vi "drive straight auto.vi"(7 "PID stuff":T1={"K Derivative"=0.000578344411839991, "K Proportional"=0.06728988505411036, "K Integral"=0.0} {"K Integral" scale=0.0..0.1; "K Proportional" scale=0.0..0.1; "K Derivative" scale=0.0..0.1}, 10 "Foward Power":dbl(knob) scale=0.0..1.0, 11 "Foward Distance":dbl) -> ()   [LabVIEW 2011]
uses:
  <vilib>/addons/control/pid/pid.llb/PID (DBL).vi
  <vilib>/addons/control/pid/NI_PID_pid.lvlib
panel:
  out "Waveform Chart":dbl(graph)
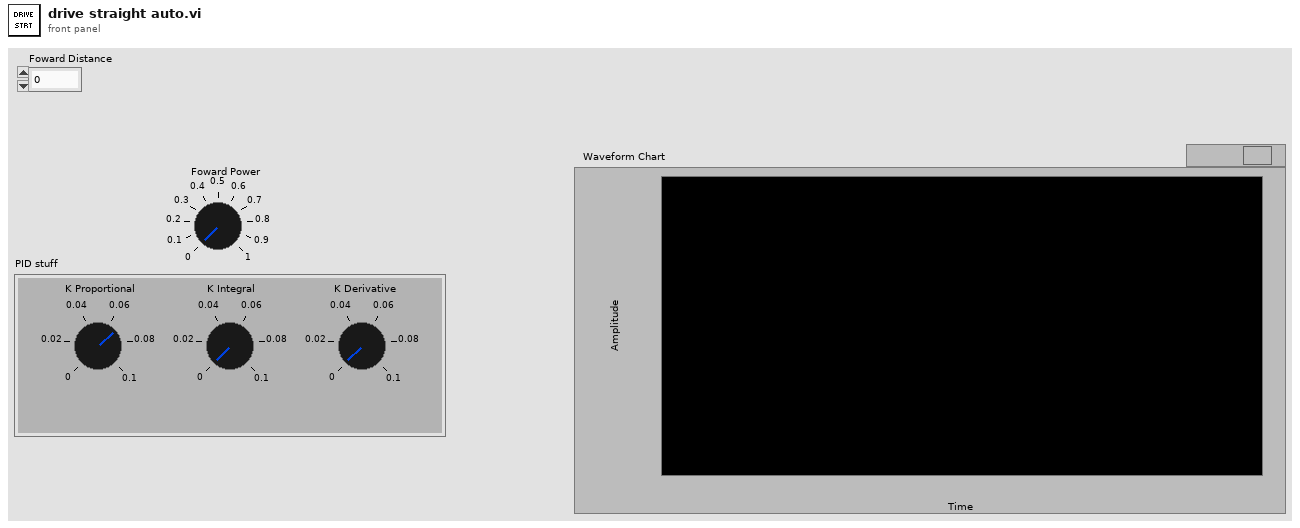
[diagram p1: front panel]
types:
  T1 = cluster{"K Derivative":dbl, "K Proportional":dbl, "K Integral":dbl}
  T2 = typedef "WPI_EncoderDevRef.ctl" = cluster{"DevStatus":errorcluster, "EncoderIndex":T3, "CounterIndex":T4, "DistancePerCount":dbl, "Decoding Type":T5}
  T3 = typedef "FPGA_EncoderIdx.ctl" = enum8{"Enc 0", "Enc 1", "Enc 2", "Enc 3", "Invalid"}
  T4 = typedef "FPGA_CounterCtrSystemIndex.ctl" = enum8{"Ctr 0", "Ctr 1", "Ctr 2", "Ctr 3", "Ctr 4", "Ctr 5", "Ctr 6", "Ctr 7", "Invalid"}
  T5 = typedef "WPI_EncoderType.ctl" = enum16{"1x", "2x", "4x"}
  T6 = typedef "WPI_GyroDevRef.ctl" = cluster{"DevStatus":errorcluster, "Analog Module":T7, "Analog Channel":T8, "Offset":dbl, "Gain (VoltsPerDegree/Second)":dbl}
  T7 = typedef "FPGA_TypedefAnalogModule.ctl" = enum16{"Analog Module 1", "Analog Module 2"}
  T8 = typedef "FPGA_AIChannel.ctl" = enum8{"AI 1", "AI 2", "AI 3", "AI 4", "AI 5", "AI 6", "AI 7", "AI 8", "Invalid"}
  T9 = typedef "WPI_RobotDriveDevRef.ctl" = cluster{"DevStatus":errorcluster, "Motors[]":T10[], "Square Inputs":bool, "Max Output":dbl, "Isochronous":bool}
  T10 = typedef "WPI_MotorControlDeviceRef.ctl" = cluster{"DeviceStatus":errorcluster, "Type":enum16{"PWM", "CAN"}, "PWM":cluster{"Digital Module":T11, "PWM Channel":T12, "DeadBand":T13}, "CAN":cluster{"Device Number":u8, "Control Mode":T14, "Semaphore":T15, "Max Vout":dbl}, "Invert":bool, "TransformRef":T16, "InvTransformRef":T16}
  T11 = typedef "FPGA_TypedefDigitalModule.ctl" = enum16{"Digital Module 1", "Digital Module 2"}
  T12 = typedef "FPGA_DIOPWMChannel.ctl" = enum8{"PWM 1", "PWM 2", "PWM 3", "PWM 4", "PWM 5", "PWM 6", "PWM 7", "PWM 8", "PWM 9", "PWM 10", "Invalid"}
  T13 = typedef "WPI_PWMDeadband.ctl" = cluster{"Name":string, "maxPositivePwm":i32, "minPositivePwm":i32, "centerPwm":i32, "maxNegativePwm":i32, "minNegativePwm":i32, "angularRange":u16}
  T14 = typedef "WPI_CANJaguar_ControlMode.ctl" = enum8{"Percent VBus", "Current", "Speed", "Position", "Voltage"}
  T15 = typedef "Semaphore RefNum" = refnum<k1>
  T16 = typedef "WPI_PWMTransform_ConPane.ctl" = refnum<vi>
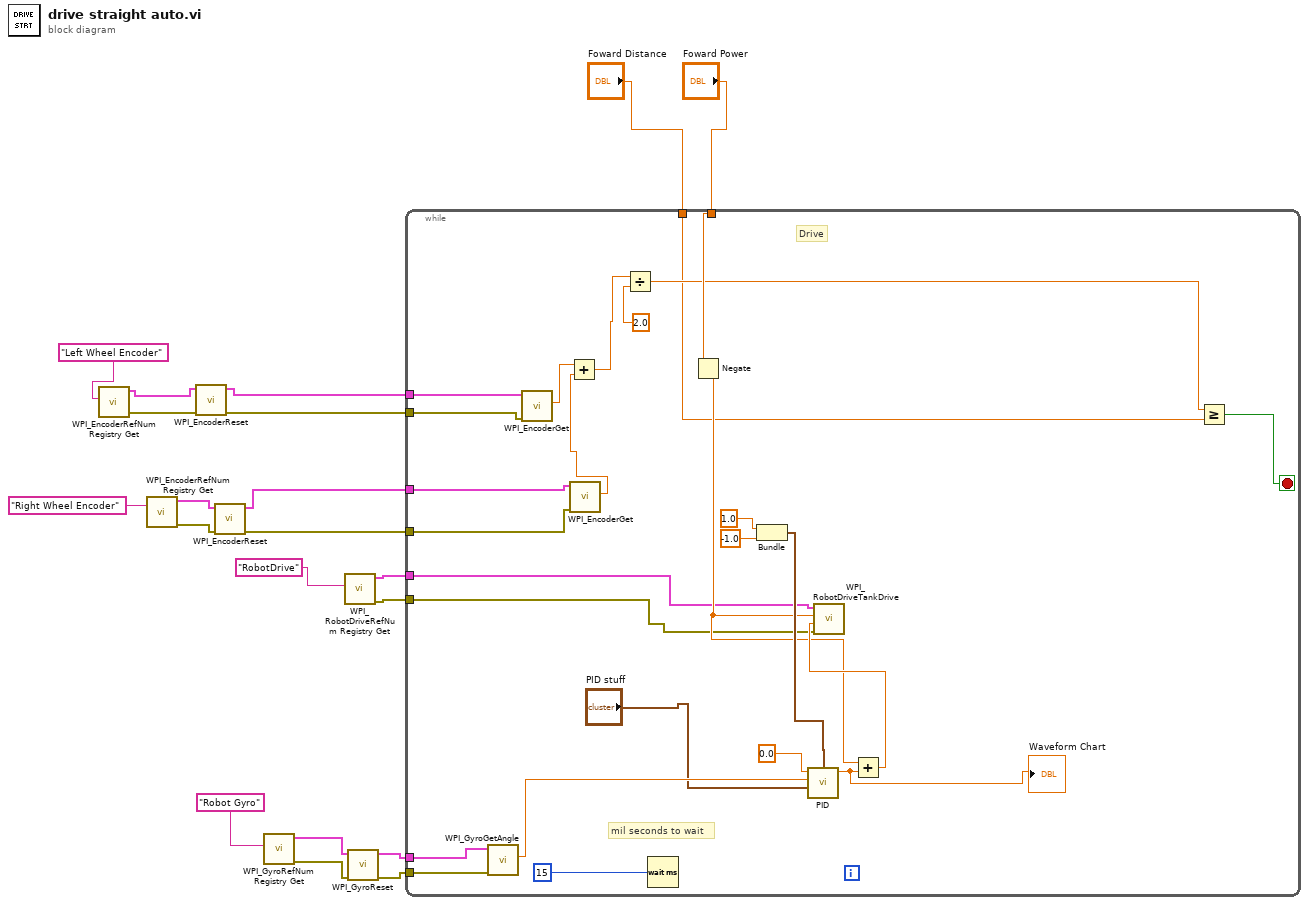
[diagram p0: block diagram]
diagram:
  n1 = call <vilib>:"WPI_EncoderRefNum Registry Get.vi"("refnum name"="Left Wheel Encoder") -> ("error out"=w16:errorcluster, "EncoderDevRef"=w17:T2)  [unwired: 9 in]
  n2 = call <vilib>:"WPI_EncoderRefNum Registry Get.vi"("refnum name"="Right Wheel Encoder") -> ("error out"=w14:errorcluster, "EncoderDevRef"=w15:T2)  [unwired: 9 in]
  n3 = call <vilib>:"WPI_EncoderReset.vi"("error in (no error)"=w16, "EncoderDevRef"=w17) -> ("error out"=w10:errorcluster, "EncoderDevRef"=w11:T2)  [unwired: 8 in]
  n4 = call <vilib>:"WPI_EncoderReset.vi"("error in (no error)"=w14, "EncoderDevRef"=w15) -> ("error out"=w12:errorcluster, "EncoderDevRef"=w13:T2)  [unwired: 8 in]
  n5 = call <vilib>:"WPI_GyroRefNum Registry Get.vi"("refnum name"="Robot Gyro") -> ("error out"=w2:errorcluster, "GyroDevRef"=w3:T6)  [unwired: 9 in]
  n6 = call <vilib>:"WPI_RobotDriveRefNum Registry Get.vi"("refnum name"="RobotDrive") -> ("error out"=w6:errorcluster, "RobotDriveDevRef"=w7:T9)  [unwired: 9 in]
  n7 = call <vilib>:"WPI_GyroReset.vi"("error in (no error)"=w2, "GyroDevRef"=w3) -> ("error out"=w5:errorcluster, "GyroDevRef"=w4:T6)  [unwired: 8 in]
  n8 = while {
    tunnel: "Foward Distance" -> [w21]
    tunnel: "Foward Power" -> [w43]
    tunnel: w13 -> [w30]
    tunnel: w12 -> [w29]
    tunnel: w11 -> [w28]
    tunnel: w10 -> [w27]
    tunnel: w4 -> [w26]
    tunnel: w5 -> [w25]
    tunnel: w7 -> [w24]
    tunnel: w6 -> [w23]
    stop <- w39 stop-if-true
    # "mil seconds to wait"
    # "Drive"
    n9 = call <vilib>:"WPI_GyroGetAngle.vi"("error in (no error)"=w25, "GyroDevRef"=w26) -> ("Angle"=w34:dbl)  [unwired: 6 in, 3 out]
    n10 = call <vilib>:"WPI_EncoderGet.vi"("error in (no error)"=w27, "EncoderDevRef"=w28) -> ("Distance"=w33:dbl)  [unwired: 4 in, 5 out]
    n11 = call <vilib>:"WPI_EncoderGet.vi"("error in (no error)"=w29, "EncoderDevRef"=w30) -> ("Distance"=w35:dbl)  [unwired: 4 in, 5 out]
    n12 = Add(x=w33, y=w35) -> (x+y=w32:dbl)
    n13 = Divide(x=w32, y=2.0) -> (x/y=w37:dbl)
    n14 = Wait (ms)(milliseconds to wait=u32 15) -> ()  [unwired: 1 out]
    n15 = Negate(x=w43) -> (-x=w36:dbl)
    n16 = Bundle(1.0, -1.0) -> (w44:cluster{dbl, dbl})  [unwired: 1 out]
    n17 = call-poly <vilib>:"PID.vi"("output range"=w44, "PID gains"="PID stuff", "process variable"=w34, "setpoint"=0.0) -> ("output"=w31:dbl)  [unwired: 2 in, 5 out]
    "Waveform Chart" <- w31
    n18 = Add(x=w36, y=w31) -> (x+y=w40:dbl)
    n19 = call <vilib>:"WPI_RobotDriveTankDrive.vi"("error in (no error)"=w23, "Right axis value"=w40, "Left axis value"=w36, "RobotDriveDevRef"=w24) -> ()  [unwired: 8 out]
    n20 = Greater Or Equal?(x=w37, y=w21) -> (x >= y?=w39:bool)
  }
